vi "Write_Instr.vi"(8 "error in (no error)":errorcluster caption="entrée d'erreur (pas d'erreur)", 11 "Class DIO en entrée":refnum<class "Class Instrument Log_File.lvclass">) -> (0 "error out":errorcluster caption="sortie d'erreur", 3 "Class DIO en Sortie":refnum<class "Class Instrument Log_File.lvclass">)   [LabVIEW 2020, in "Library Instrument & Equipement.lvlib" / "Library Instruments.lvlib" / "Class Instrument Log_File.lvclass"]
uses:
  Class Instrument Log_File.lvclass
  Class Instrument Log_File.lvclass/Class Instrument Log_File.ctl
  Instrument (Default)/Class Instrument (Default).lvclass
  Log File/Class Log_File Altyor/Class Log_File Altyor.lvclass
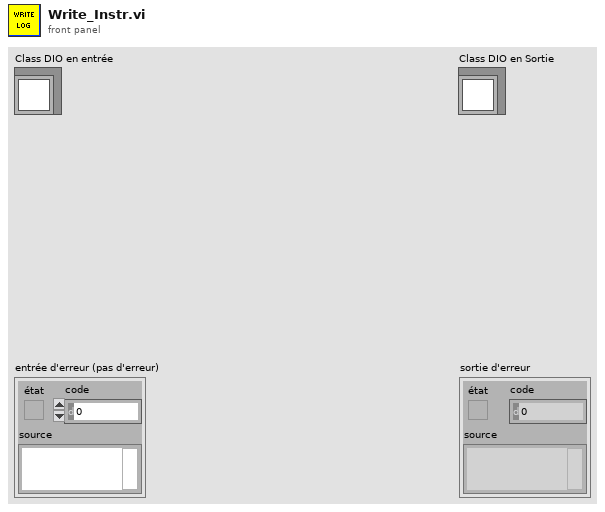
[diagram p1: front panel]
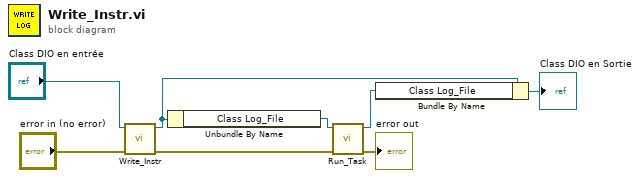
[diagram p0: block diagram]
diagram:
  n1 = call-parent "Write_Instr.vi"("error in (no error)"="error in (no error)", "Class Multimeter (Default) en entrée"="Class DIO en entrée") -> ("error out"=w3:errorcluster, "Class Multimeter (Default) en sortie"=w6:refnum<class "Class Instrument Log_File.lvclass">)  [unwired: 8 in]
  n2 = Unbundle By Name(w6) -> ("Class Log_File"=w4:refnum<class "Class Log_File Altyor.lvclass">)
  n3 = call-dynamic "Run_Task.vi"("error in (no error)"=w3, "Class Log_File Altyor en entrée"=w4) -> ("error out"=→"error out":errorcluster, "Class Log_File Altyor en sortie"=w1:refnum<class "Class Log_File Altyor.lvclass">)  [unwired: 8 in]
  n4 = Bundle By Name(cluster=w6, "Class Log_File"=w1) -> (→"Class DIO en Sortie":refnum<class "Class Instrument Log_File.lvclass">)
